vi "Create from Raw Data.vi"(7 "Endpoint":refnum<class "Endpoint.lvclass">, 8 "error in (no error)":errorcluster, 11 "Raw Data":string) -> (0 "error out":errorcluster, 3 "Message out":refnum<class "Message.lvclass">)   [LabVIEW 2020, in "Stream-Simple-Msg.lvlib" / "Message.lvclass"]
uses:
  Message.lvclass
  Endpoint/Endpoint.lvclass
  Message Data.ctl
  Message.lvclass/Message.ctl
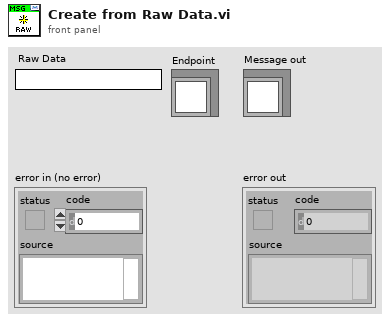
[diagram p1: front panel]
types:
  T1 = typedef "Stream-Simple-Msg.lvlib/Message.lvclass/Message Data.ctl" = cluster{"ID":string, "Data":string}
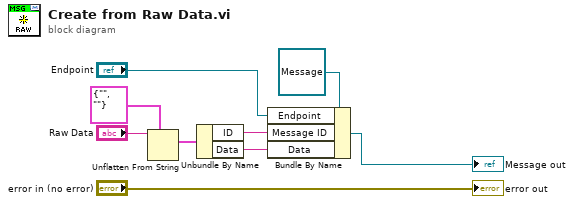
[diagram p0: block diagram]
diagram:
  n1 = Unflatten From String(type=T1 {"ID"="", "Data"=""} ("Message Data"), binary string="Raw Data") -> (value=w5:T1)  [unwired: 3 in, 2 out]
  n2 = Unbundle By Name(w5) -> ("ID"=w3:string, "Data"=w2:string)
  n3 = Bundle By Name(cluster=refnum<class "Message.lvclass"> refnum ("Message in"), "Endpoint"="Endpoint", "Message ID"=w3, "Data"=w2) -> (→"Message out":refnum<class "Message.lvclass">)
  "error out" <- "error in (no error)"
